vi "Configuracion.vi"() -> ()   [LabVIEW 2018]
uses:
  <vilib>/RAFA Solutions/Harmony UI Controls Kit/Boolean/Blank Button - Red.ctl
  <vilib>/RAFA Solutions/Harmony UI Controls Kit/Boolean/Blank Button - Blue.ctl
  <vilib>/RAFA Solutions/Harmony UI Controls Kit/Flat UI Design.lvlib
panel:
  in  "tamaño bd":T1
  in  "modifica equipos":T1
  in  "usuarios":T1
  in  "type specifier VI Refnum (for type only) 11":refnum<vi>
  in  "SALIR":T2
  # "CONFIGURACIÓN"
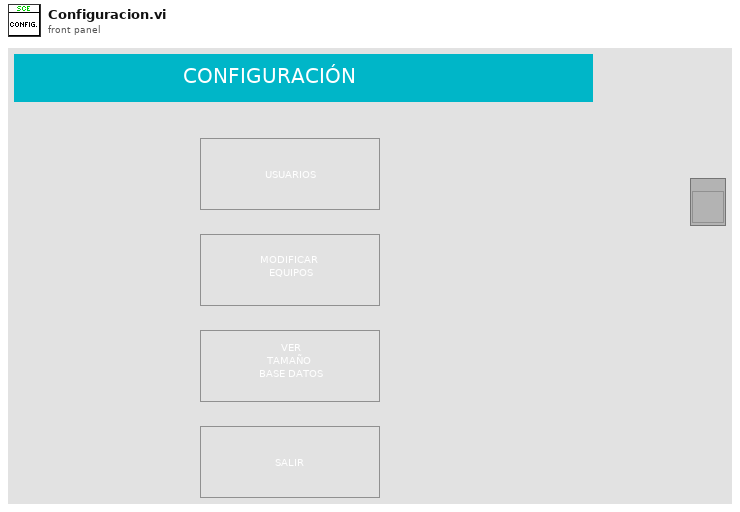
[diagram p1: front panel]
types:
  T1 = typedef "Flat UI Design.lvlib/Blank Button - Blue.ctl" = bool
  T2 = typedef "Flat UI Design.lvlib/Blank Button - Red.ctl" = bool
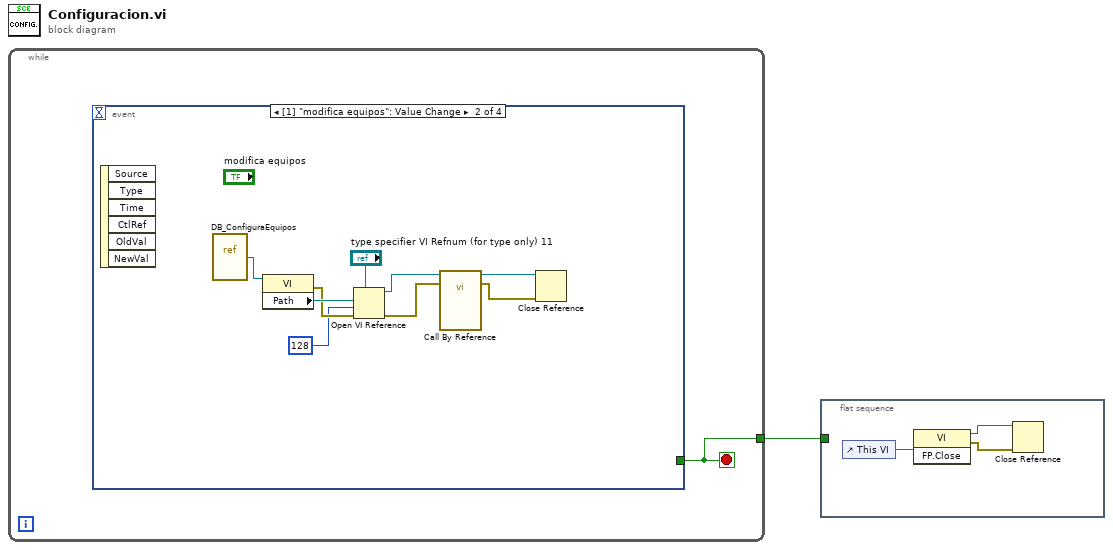
[diagram p0: block diagram]
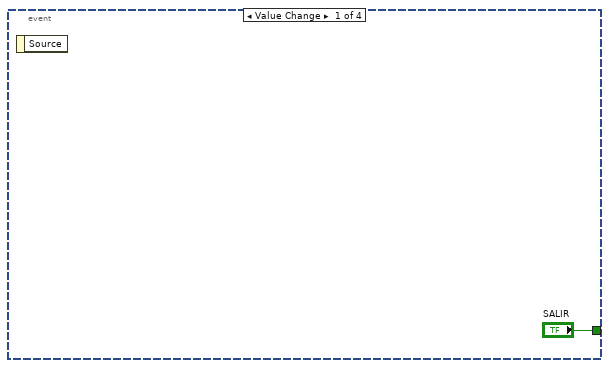
[diagram p2: hidden frame]
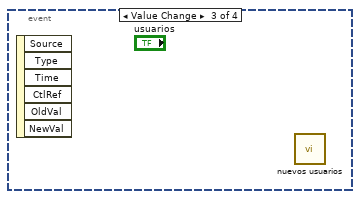
[diagram p3: hidden frame]
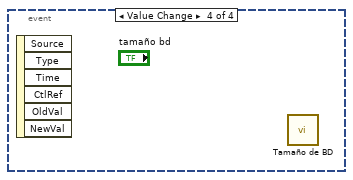
[diagram p4: hidden frame]
diagram:
  n1 = while {
    tunnel: [w2] -> w1
    stop <- w2 stop-if-true
    n2 = event shown="[1] \"modifica equipos\": Value Change" {
      selector: _ -> [_ _ _ _]
      dyn-events: _ -> [_ _ _ _]
      timeout: _ -> [_ _ _ _]
      tunnel: ["SALIR" _ _ _] -> w2
      event Value Change {
        n3 = event-data() -> ()  [unwired: 1 in, 1 out]
      }
      event Value Change {
        n4 = event-data() -> ()  [unwired: 1 in, 6 out]
        n5 = vi-ref "DB_ConfiguraEquipos.vi"() -> (w7:refnum<vi>)
        n6 = property class="VI"(reference=w7) -> (error out=w5:errorcluster, "Path"=w6:path)  [unwired: 1 in, 1 out]
        n7 = Open VI Reference(type specifier VI Refnum (for type only)="type specifier VI Refnum (for type only) 11", vi path=w6, options=128, error in (no error)=w5) -> (vi reference=w8:refnum<vi>, error out=w12:errorcluster)  [unwired: 2 in]
        n8 = call-by-ref "?"(reference=w8, error in=w12) -> (reference out=w11:refnum<vi>, error out=w10:errorcluster)  [unwired: 12 in]
        n9 = Close Reference(reference=w11, error in (no error)=w10) -> ()  [unwired: 1 out]
      }
      event Value Change {
        n10 = event-data() -> ()  [unwired: 1 in, 6 out]
        n11 = call "nuevos usuarios.vi"() -> ()  [unwired: 12 in]
      }
      event Value Change {
        n12 = event-data() -> ()  [unwired: 1 in, 6 out]
        n13 = call "Tamaño de BD.vi"() -> ()  [unwired: 12 in]
      }
    }
  }
  n14 = flat-sequence {
    tunnel: w1 -> [_]
    frame #0 {
      n15 = control-ref of="This VI"() -> (w15:refnum<vi>)
      n16 = invoke class="VI" method="FP.Close"(reference=w15) -> (reference out=w14:refnum<vi>, error out=w13:errorcluster)  [unwired: 2 in, 1 out]
      n17 = Close Reference(reference=w14, error in (no error)=w13) -> ()  [unwired: 1 out]
    }
  }
